vi "Create Channel Array.vi"(8 "error in":errorcluster, 10 "channel settings":T1[](array[typedef]), 11 "analog input mode in":refnum<class "Analog Input Mode.lvclass">) -> (0 "error out":errorcluster, 2 "channels":refnum<class "AI Channel.lvclass">[](array[class]), 3 "analog input mode out":refnum<class "Analog Input Mode.lvclass">)   [LabVIEW 2020, in "Scan Engine Scripting.lvlib" / "Analog Input Mode.lvclass"]
uses:
  Analog Input Mode.lvclass
  Controls/analog channel settings.ctl
  Channel Classes/AI Channel/AI Channel.lvclass
  Scan Engine Scripting.lvlib
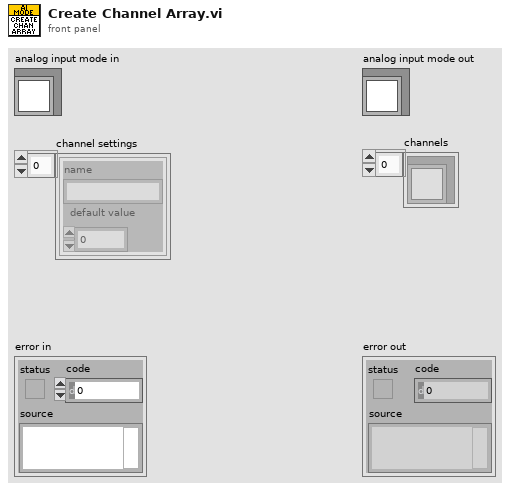
[diagram p1: front panel]
types:
  T1 = typedef "Scan Engine Scripting.lvlib/analog channel settings.ctl" = cluster{"name":string, "default value":dbl}
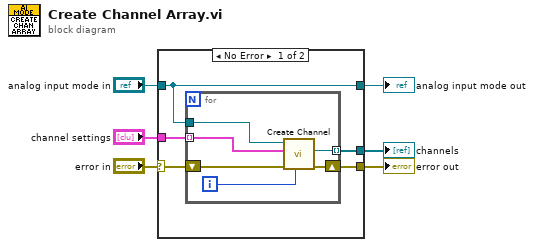
[diagram p0: block diagram]
diagram:
  n1 = case shown="No Error" "error in" {
    selector: "error in" -> [w10 w19]
    tunnel: [w7 w19] -> w5
    tunnel: [w9 w18] -> w3
    tunnel: "analog input mode in" -> [w9 w18]
    tunnel: "channel settings" -> [w11 _]
    tunnel: [w8 _] -> w1
    frame No Error {
      n2 = for {
        tunnel: w11 -> [w12] mode=indexing
        shift-right: [w15] -> w7
        shift-left: w10 -> [w16]
        tunnel: [w14] -> w8 mode=indexing
        tunnel: w9 -> [w17]
        i -> [w13]
        n3 = call "Create Channel.vi"("index"=w13, "error in"=w16, "channel settings"=w12, "analog input mode in"=w17) -> ("error out"=w15:errorcluster, "analog input channel"=w14:refnum<class "AI Channel.lvclass">)  [unwired: 5 in, 1 out]
      }
    }
    frame Error {
    }
  }
  "error out" <- w5
  "analog input mode out" <- w3
  "channels" <- w1
